vi "Rotation Control.vi"(10 "Prior Mode":T1, 11 "Color Sensor Input":string) -> (3 "Done":bool)   [LabVIEW 2019]
uses:
  Vanna Mode Type Def.ctl
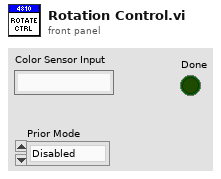
[diagram p1: front panel]
types:
  T1 = typedef "Vanna Mode Type Def.ctl" = enum16{"Disabled", "Raw Throttle", "Rotation Control", "Position Control"}
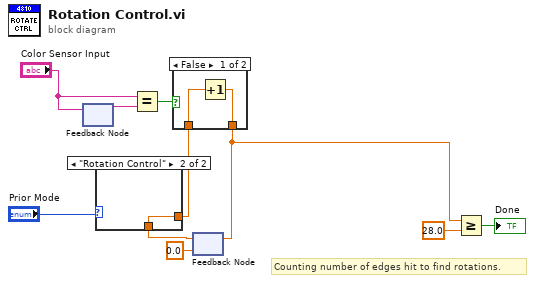
[diagram p0: block diagram]
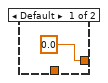
[diagram p2: hidden frame]
diagram:
  # "Counting number of edges hit to find rotations."
  n1 = feedback-in #1("Color Sensor Input") -> ()
  n2 = feedback #1() -> (w10:string)  [unwired: 1 in]
  n3 = Equal?(x="Color Sensor Input", y=w10) -> (x = y?=w8:bool)
  n4 = feedback #2(0.0) -> (w2:dbl)
  n5 = case shown="\"Rotation Control\"" "Prior Mode" {
    tunnel: w2 -> [_ w12]
    tunnel: [0.0 w12] -> w1
    frame Default {
    }
    frame "Rotation Control" {
    }
  }
  n6 = case shown="False" w8 {
    tunnel: [w14 w15] -> w3
    tunnel: w1 -> [w13 w15]
    frame False {
      n7 = Increment(x=w13) -> (x+1=w14:dbl)
    }
    frame True {
    }
  }
  n8 = feedback-in #2(w3) -> ()
  n9 = Greater Or Equal?(x=w3, y=28.0) -> (x >= y?=→"Done":bool)
